vi "Render.vi"(7 "Renderer":refnum<class "Renderer.lvclass">, 8 "error in (no error)":errorcluster, 10 "Camera":refnum<class "Camera.lvclass">, 11 "Zap Sat in":refnum<class "Zap Sat.lvclass">) -> (0 "error out":errorcluster)   [LabVIEW 2021, in "Zap Sat.lvclass"]
uses:
  Zap Sat.lvclass
  Camera/Camera.lvclass
  Renderer/Renderer.lvclass
  Zap Sat.lvclass/Zap Sat.ctl
  Re-use Libraries/Vector 2D/Vector 2D.lvclass
  Element/Element.lvclass
  Deployable/Deployable.lvclass
  Resource Manager/Resource Manager.lvclass
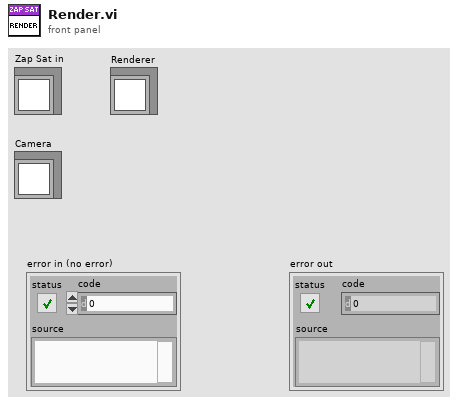
[diagram p1: front panel]
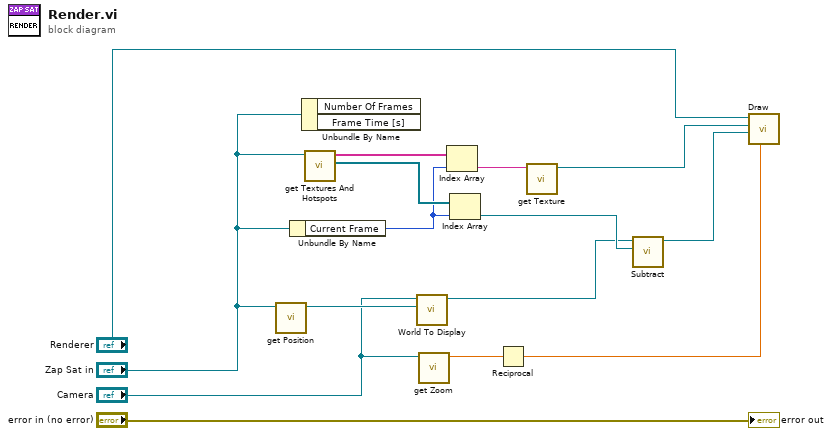
[diagram p0: block diagram]
diagram:
  n1 = call "get Position.vi"("Element in"="Zap Sat in") -> ("Position"=w14:refnum<class "Vector 2D.lvclass">)  [unwired: 10 in]
  n2 = Unbundle By Name("Zap Sat in") -> ("Current Frame"=w5:i32)
  n3 = Unbundle By Name("Zap Sat in") -> ()  [unwired: 2 out]
  n4 = call "get Textures And Hotspots.vi"("Deployable in"="Zap Sat in") -> ("Hotspots"=w6:refnum<class "Vector 2D.lvclass">[], "Textures"=w9:string[])  [unwired: 9 in]
  n5 = call "World To Display.vi"("World Position"=w14, "Camera in"="Camera") -> ("Display Position"=w1:refnum<class "Vector 2D.lvclass">)  [unwired: 9 in]
  n6 = call "get Zoom.vi"("Camera in"="Camera") -> ("Zoom Level"=w15:sgl)  [unwired: 10 in]
  n7 = Index Array(array=w9, index=w5) -> (element=w8:string)
  n8 = Index Array(array=w6, index=w5) -> (element=w4:refnum<class "Vector 2D.lvclass">)
  n9 = Reciprocal(x=w15) -> (1/x=w12:sgl)
  n10 = call "get Texture.vi"("Texture Name"=w8) -> ("Texture"=w7:refnum<class "Texture.lvclass">)  [unwired: 10 in]
  n11 = call "Subtract.vi"("B"=w4, "A"=w1) -> ("A-B"=w3:refnum<class "Vector 2D.lvclass">)  [unwired: 9 in]
  n12 = call "Draw.vi"("Scale"=w12, "Destination"=w3, "Texture"=w7, "Renderer"="Renderer") -> ()  [unwired: 7 in, 1 out]
  "error out" <- "error in (no error)"
